vi "Init.vi"(8 "error in (no error)":errorcluster, 11 "reference in":refnum<class "DUT_Handler_Base.lvclass">) -> (0 "error out":errorcluster, 3 "reference out":refnum<class "DUT_Handler_Base.lvclass">)   [LabVIEW 2022 SP3, in "DUT_Handler_Base.lvlib" / "DUT_Handler_Base.lvclass"]
uses:
  DUT_Handler_Base.lvclass
  EventData.ctl
  Action.ctl
  Components/ViPER.lvlibp/ViPER.lvclass
  C:/Projects/Medulla/ViPER/Examples/Flux_Capacitor_Tester/Components/ViPER.lvlibp/ViPER.lvclass
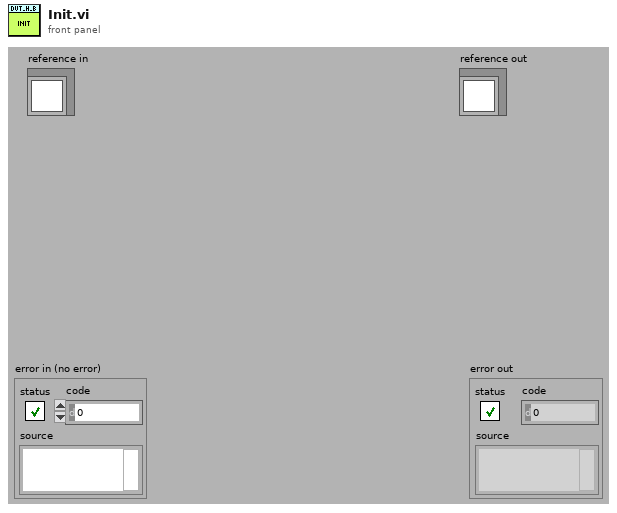
[diagram p1: front panel]
types:
  T1 = typedef "DUT_Handler_Base.lvlib/DUT_Handler_Base.lvclass/EventData.ctl" = cluster{"Action":T2, "SN":string, "BN":string, "DUT__ID":u32, "Message":string, "From":string, "To":string}
  T2 = typedef "DUT_Handler_Base.lvlib/DUT_Handler_Base.lvclass/Action.ctl" = enum16{"Load", "Cancel", "MoveIn", "MoveOut", "Abort", "Msg", "Enabled", "Disabled", "Fault", "Shutdown"}
  T3 = typedef "DUT_Handler_Base.lvlib/DUT_Handler_Base.lvclass/ObjectAttributes.ctl" = cluster{"Config":T4, "Event":refnum<user-event>}
  T4 = typedef "DUT_Handler_Base.lvlib/DUT_Handler_Base.lvclass/Config.ctl" = cluster{"default":string}
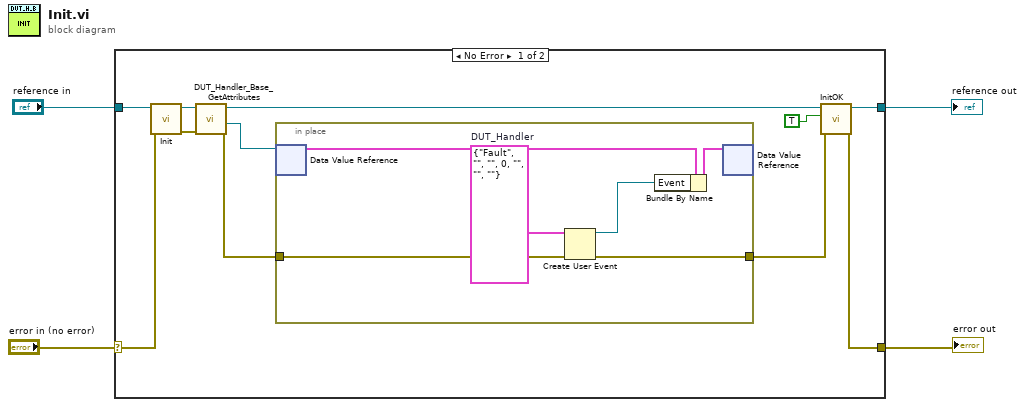
[diagram p0: block diagram]
diagram:
  n1 = case shown="No Error" "error in (no error)" {
    selector: "error in (no error)" -> [w14 w23]
    tunnel: [w5 w23] -> w3
    tunnel: [w8 w22] -> w1
    tunnel: "reference in" -> [w15 w22]
    frame No Error {
      n2 = call-parent "Init.vi"("error in (no error)"=w14, "reference in"=w15) -> ("error out"=w12:errorcluster, "reference out"=w13:refnum<class "DUT_Handler_Base.lvclass">)  [unwired: 8 in]
      n3 = call "DUT_Handler_Base_GetAttributes.vi"("error in (no error)"=w12, "reference in"=w13) -> ("error out"=w10:errorcluster, "DataRef"=w11:refnum<data-value>, "reference out"=w9:refnum<class "DUT_Handler_Base.lvclass">)  [unwired: 6 in, 1 out]
      n4 = in-place {
        in-place-border: w10 -> [w21]
        in-place-border: [w20] -> w6
        w19 = T1 {"Action"=enum."Fault", "SN"="", "BN"="", "DUT__ID"=0, "Message"="", "From"="", "To"=""}  # DUT_Handler
        n5 = in-place-dvr #1(w11) -> (w18:T3)  [unwired: 1 out]
        n6 = Create User Event(user event datatype=w19, error in=w21) -> (user event=w16:refnum<user-event>, error out=w20:errorcluster)
        n7 = Bundle By Name(cluster=w18, "Event"=w16) -> (w17:T3)
        n8 = in-place-dvr #1(w17) -> ()  [unwired: 2 out]
      }
      n9 = call "InitOK.vi"("error in (no error)"=w6, "Init OK?"=TRUE, "reference in"=w9) -> ("error out"=w5:errorcluster, "reference out"=w8:refnum<class "DUT_Handler_Base.lvclass">)  [unwired: 7 in]
    }
    frame Error {
    }
  }
  "error out" <- w3
  "reference out" <- w1
